vi "Write Data.vi"(8 "error in":errorcluster, 10 "PAS Data.lvclass":refnum<class "PAS Data.lvclass">, 11 "PAS in":refnum<class "PAS.lvclass">) -> (0 "error out":errorcluster, 3 "PAS out":refnum<class "PAS.lvclass">)   [LabVIEW 2015, in "PAS.lvclass"]
uses:
  PAS.lvclass
  Data/Main/PAS Data.lvclass
  PAS.lvclass/PAS.ctl
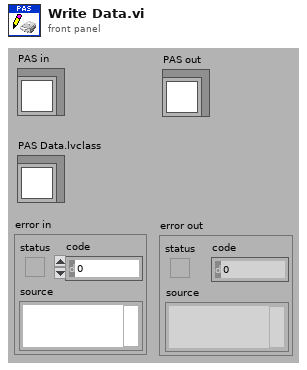
[diagram p1: front panel]
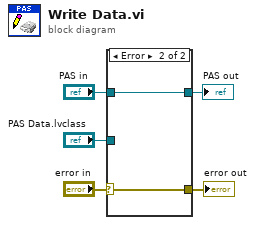
[diagram p0: block diagram]
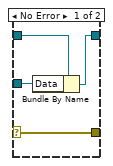
[diagram p2: hidden frame]
diagram:
  n1 = case shown="Error" "error in" {
    selector: "error in" -> [w6 w10]
    tunnel: "PAS in" -> [w9 w11]
    tunnel: [w8 w11] -> w4
    tunnel: "PAS Data.lvclass" -> [w7 _]
    tunnel: [w6 w10] -> w1
    frame No Error {
      n2 = Bundle By Name(cluster=w9, "Data"=w7) -> (w8:refnum<class "PAS.lvclass">)
    }
    frame Error {
    }
  }
  "error out" <- w1
  "PAS out" <- w4
